vi "ma_Initial guess for tone estimation (amplitude input).vi"(2 "spectral info":T1 {"window" items=["Rectangle"=0, "Hanning"=1, "Hamming"=2, "Blackman-Harris"=3, "Exact Blackman"=4, "Blackman"=5, "Flat Top"=6, "4 Term B-Harris "=7, "7 Term B-Harris"=8, "Low Sidelobe"=9, "Blackman Nuttall"=11, "Triangle"=30, "Bartlett-Hanning"=31, "Bohman"=32, "Parzen"=33, "Welch"=34, "Kaiser"=60, "Dolph-Chebyshev"=61, "Gaussian"=62]}, 3 "three fingers":T2={"f0"=0.0, "df"=1.0, "spectrum"=[]} {"spectrum" format="%.2f"; "df" format="%.2f"; "f0" format="%.2f"}) -> (0 "range":cluster{"f upper":dbl, "f lower":dbl} {"f lower" format="%.2e"; "f upper" format="%.2e"}, 1 "initial guess frequecy":dbl format="%.9f")   [LabVIEW 2020, in "NI_MAPro.lvlib"]
uses:
  NI_MAPro.lvlib
  ma_sml_Spectrum Cluster (real).ctl
  ma_sml_Spectral Info.ctl
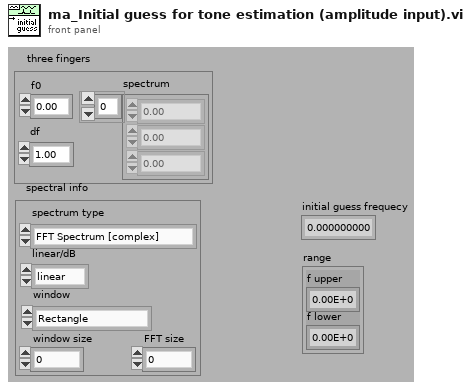
[diagram p1: front panel]
types:
  T1 = typedef "NI_MAPro.lvlib/ma_sml_Spectral Info.ctl" = cluster{"spectrum type":enum16{"FFT Spectrum [complex]", "Amplitude [Magnitude]", "Power [Magnitude^2]", "Cross Spectrum [complex]", "Frequency Response [Complex]"}, "linear/dB":enum16{"linear", "dB"}, "window":u16, "window size":i32, "FFT size":i32}
  T2 = typedef "NI_MAPro.lvlib/ma_sml_Spectrum Cluster (real).ctl" = cluster{"f0":dbl, "df":dbl, "spectrum":dbl[]}
  T3 = enum16{"None ", "Hanning", "Hamming", "Blackman-Harris", "Exact Blackman", "Blackman", "Flat Top", "4 Term B-Harris ", "7 Term B-Harris", "Low Sidelobe"}
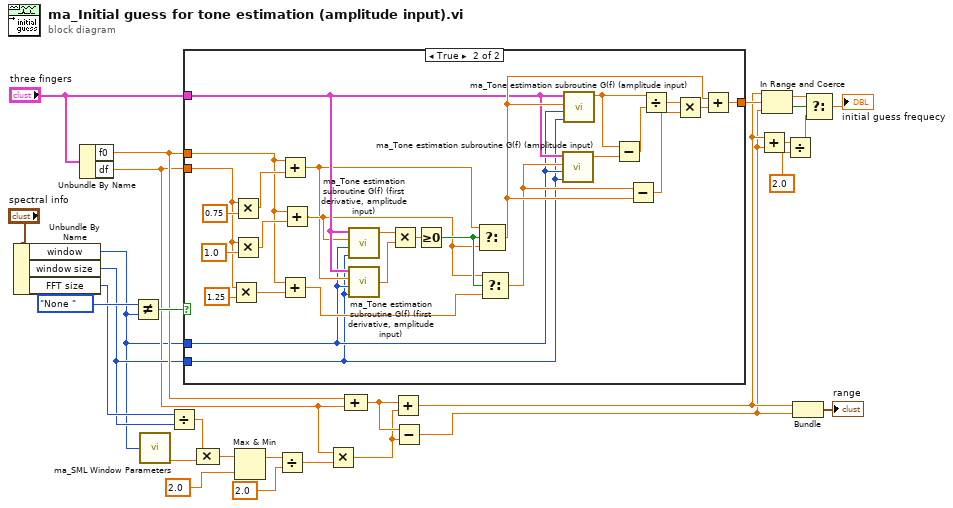
[diagram p0: block diagram]
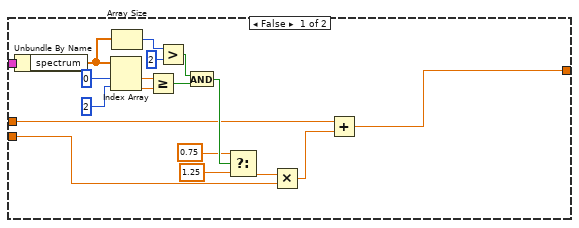
[diagram p2: hidden frame]
diagram:
  n1 = Unbundle By Name("spectral info") -> ("window"=w2:u16, "window size"=w13:i32, "FFT size"=w14:i32)
  n2 = Unbundle By Name("three fingers") -> ("f0"=w19:dbl, "df"=w11:dbl)
  n3 = Not Equal?(x=T3."None " ("window"), y=w2) -> (x != y?=w26:bool)
  n4 = call "ma_SML Window Parameters.vi"("window"=w2) -> ("6dB BW"=w1:dbl)  [unwired: 3 out]
  n5 = Divide(x=w14, y=w13) -> (x/y=w16:dbl)
  n6 = case shown="True" w26 {
    tunnel: [w45 w66] -> w28
    tunnel: "three fingers" -> [w34 w56]
    tunnel: w19 -> [w29 w55]
    tunnel: w11 -> [w30 w54]
    tunnel: w2 -> [_ w48]
    tunnel: w13 -> [_ w47]
    frame False {
      n7 = Unbundle By Name(w34) -> ("spectrum"=w31:dbl[])
      n8 = Index Array(array=w31, index #1=0 ("Index"), index #2=2 ("Index")) -> (element #1=w33:dbl, element #2=w32:dbl)
      n9 = Array Size(array=w31) -> (size(s)=w39:i32)
      n10 = Greater Or Equal?(x=w33, y=w32) -> (x >= y?=w42:bool)
      n11 = Greater?(x=w39, y=2) -> (0:w37:bool)
      n12 = And(x=w37, y=w42) -> (x .and. y?=w40:bool)
      n13 = Select(t=0.75 ("x"), s=w40, f=1.25) -> (s? t:f=w41:dbl)
      n14 = Multiply(x=w41, y=w30) -> (x*y=w46:dbl)
      n15 = Add(x=w29, y=w46) -> (x+y=w45:dbl)
    }
    frame True {
      n16 = Multiply(x=w54, y=1.25 ("f")) -> (x*y=w61:dbl)
      n17 = Multiply(x=w54, y=0.75 ("t")) -> (x*y=w72:dbl)
      n18 = Multiply(x=w54, y=1.0 ("f")) -> (x*y=w71:dbl)
      n19 = Add(x=w55, y=w72) -> (x+y=w49:dbl)
      n20 = Add(x=w55, y=w61) -> (x+y=w50:dbl)
      n21 = Add(x=w55, y=w71) -> (x+y=w51:dbl)
      n22 = call "ma_Tone estimation subroutine G(f) (first derivative, amplitude input).vi"("N (window length)"=w47, "window"=w48, "frequency"=w51, "three fingers"=w56) -> ("G'(f)"=w53:dbl)
      n23 = call "ma_Tone estimation subroutine G(f) (first derivative, amplitude input).vi"("N (window length)"=w47, "window"=w48, "frequency"=w49, "three fingers"=w56) -> ("G'(f)"=w52:dbl)
      n24 = Multiply(x=w53, y=w52) -> (x*y=w60:dbl)
      n25 = Greater Or Equal To 0?(x=w60) -> (x >= 0?=w59:bool)
      n26 = Select(t=w49, s=w59, f=w51) -> (s? t:f=w58:dbl)
      n27 = Select(t=w51, s=w59, f=w50) -> (s? t:f=w57:dbl)
      n28 = call "ma_Tone estimation subroutine G(f) (amplitude input).vi"("N (window length)"=w47, "window"=w48, "frequency"=w57, "three fingers"=w56) -> ("G(f)"=w69:dbl)  [unwired: 2 in, 1 out]
      n29 = call "ma_Tone estimation subroutine G(f) (amplitude input).vi"("N (window length)"=w47, "window"=w48, "frequency"=w58, "three fingers"=w56) -> ("G(f)"=w65:dbl)  [unwired: 2 in, 1 out]
      n30 = Subtract(x=w65, y=w69) -> (x-y=w70:dbl)
      n31 = Subtract(x=w57, y=w58) -> (x-y=w64:dbl)
      n32 = Divide(x=w65, y=w70) -> (x/y=w68:dbl)
      n33 = Multiply(x=w68, y=w64) -> (x*y=w67:dbl)
      n34 = Add(x=w58, y=w67) -> (x+y=w66:dbl)
    }
  }
  n35 = Compound Arithmetic op=MULTIPLY(w16, w1) -> (w17:dbl)
  n36 = Max & Min(x=w17, y=2.0) -> (max(x,y)=w22:dbl)  [unwired: 1 out]
  n37 = Divide(x=w22, y=2.0) -> (x/y=w23:dbl)
  n38 = Multiply(x=w11, y=w23) -> (x*y=w12:dbl)
  n39 = Compound Arithmetic op=ADD(w19, w11) -> (w24:dbl)
  n40 = Add(x=w24, y=w12) -> (x+y=w7:dbl)
  n41 = Subtract(x=w24, y=w12) -> (x-y=w6:dbl)
  n42 = Add(x=w7, y=w6) -> (x+y=w5:dbl)
  n43 = In Range and Coerce(upper limit=w7, x=w28, lower limit=w6) -> (coerced(x)=w10:dbl, In Range?=w8:bool)
  n44 = Divide(x=w5, y=2.0) -> (x/y=w4:dbl)
  n45 = Bundle(w7, w6) -> (→"range":cluster{dbl, dbl})  [unwired: 1 out]
  n46 = Select(t=w10, s=w8, f=w4) -> (s? t:f=→"initial guess frequecy":dbl)
